vi "Tools_String Tokenize String (Simple).vi"(4 "delimiter ([\\s\\t\\n\\r]+)":string="[ \t\n\r]+", 5 "input string":string) -> (0 "token array":string[](array[string]), 2 "number of tokens":i32)   [LabVIEW 2017]
doc: "Separates input string into an array of substrings. Delimiter specifies what separates the substrings.\n\nExample:\ndelimiter=\"[ ]+\" (i.e. one or more spaces)\ninput string= \"hello world foo\\ bar\"\n\ntoken array=[\"hello\",\"world\",\"foo\\\", \"bar\"]"
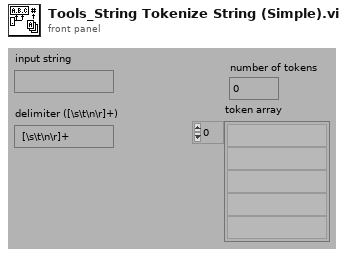
[diagram p1: front panel]
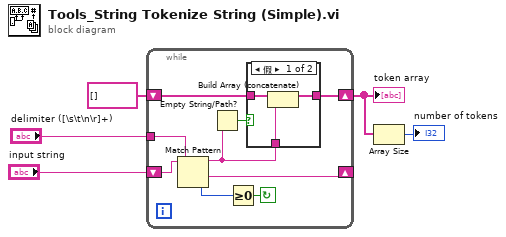
[diagram p0: block diagram]
diagram:
  n1 = while {
    shift-left: string[] [] -> [w8]
    shift-right: [w7] -> w2
    shift-left: "input string" -> [w11]
    shift-right: [w10] -> _
    tunnel: "delimiter ([\\s\\t\\n\\r]+)" -> [w14]
    stop <- w12 continue-if-true
    n2 = Match Pattern(string=w11, regular expression=w14) -> (before substring=w6:string, after substring=w10:string, offset past match=w13:i32)  [unwired: 2 out]
    n3 = Empty String/Path?(string/path=w6) -> (empty?=w9:bool)
    n4 = Greater Or Equal To 0?(x=w13) -> (x >= 0?=w12:bool)
    n5 = case shown="假" w9 {
      tunnel: w8 -> [w17 w18]
      tunnel: [w16 w18] -> w7
      tunnel: w6 -> [w15 _]
      frame False {
        n6 = Build Array (concatenate)(w17, w15) -> (w16:string[])
      }
      frame True {
      }
    }
  }
  "token array" <- w2
  n7 = Array Size(array=w2) -> (size(s)=→"number of tokens":i32)
